vi "Write Top Level Value.vi"(7 "Key":string, 8 "error in (no error)":errorcluster, 10 "Value":variant, 11 "file path (use dialog)":path) -> (0 "error out":errorcluster)   [LabVIEW 2020, in "TOML.lvlib"]
uses:
  TOML.lvlib
  LabVIEW to TOML.vi
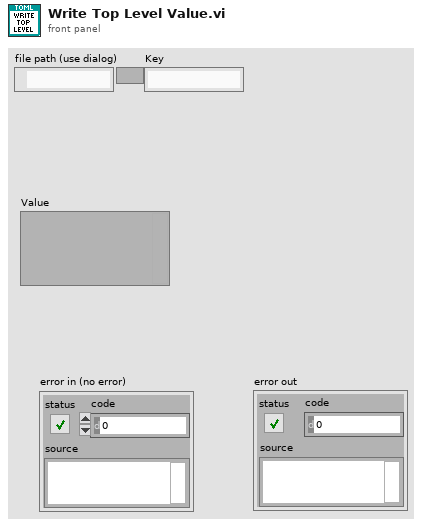
[diagram p1: front panel]
types:
  T1 = enum16{"open", "replace", "create", "open or create", "replace or create", "replace or create with confirmation"}
  T2 = typedef "TOML.lvlib/TOML Value.ctl" = cluster{"type":enum16{"Table", "Array", "String", "Integer", "Float", "Boolean", "Offset Date-Time", "Local Date-Time", "Local Date", "Local Time", "Path"}, "value":variant}
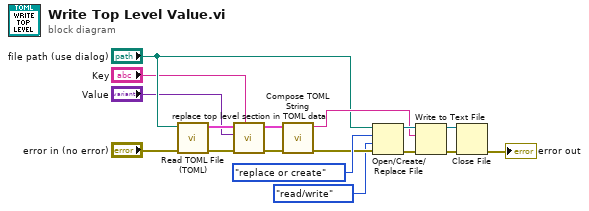
[diagram p0: block diagram]
diagram:
  n1 = call "Read TOML File (TOML).vi"("error in (no error)"="error in (no error)", "file path (use dialog)"="file path (use dialog)") -> ("error out"=w6:errorcluster, "Value"=w8:T2)  [unwired: 8 in]
  n2 = call "replace top level section in TOML data.vi"("Section name"="Key", "error in (no error)"=w6, "Section data"="Value", "Value in"=w8) -> ("error out"=w5:errorcluster, "Value out"=w7:T2)  [unwired: 6 in]
  n3 = call "Compose TOML String.vi"("error in (no error)"=w5, "Value"=w7) -> ("error out"=w10:errorcluster, "String"=w11:string)  [unwired: 8 in]
  n4 = Open/Create/Replace File(file path (use dialog)="file path (use dialog)", error in=w10, operation (0:open)=T1."replace or create", access (0:read/write)=enum16{"read/write", "read-only", "write-only"}."read/write") -> (refnum out=w15:refnum<file>, error out=w16:errorcluster)  [unwired: 2 in, 1 out]
  n5 = Write to Text File(file (use dialog)=w15, text=w11, error in=w16) -> (refnum out=w13:refnum<file>, error out=w14:errorcluster)  [unwired: 1 in, 1 out]
  n6 = Close File(refnum=w13, error in=w14) -> (error out=→"error out":errorcluster)  [unwired: 1 out]
